vi "Draw Markers.vi"(7 "XYGraph in":refnum<vi>, 9 "Marker Options":T3={"Color"=16723218, "pen"={"Width"=2, "Style"=enum."Solid"}, "font"={"Font Name"="Arial", "Size"=16, "Strikeout?"=FALSE, "Italic?"=FALSE, "Underline?"=FALSE, "Outline?"=FALSE, "Shadow?"=FALSE, "Bold?"=FALSE, "FontColor"=0}, "caption"=""}, 10 "Marker":T1={"Type"=enum."vert", "X"=2.0, "Y"=2.0, "X2"=2.0, "Y2"=2.0, "Text"="Drag and click to\nposition a marker"}, 11 "picture":picture) -> (3 "new picture":picture)   [LabVIEW 2014, in "Graph Extensions.lvlib"]
doc: "Draw the appropriate line for markers, depending on the type"
uses:
  Graph Extensions.lvlib
  <vilib>/Utility/miscctls.llb/LVPoint32TypeDef.ctl
  controls/MarkerInfo.ctl
  controls/MarkerOptions.ctl
  controls/markerType.ctl
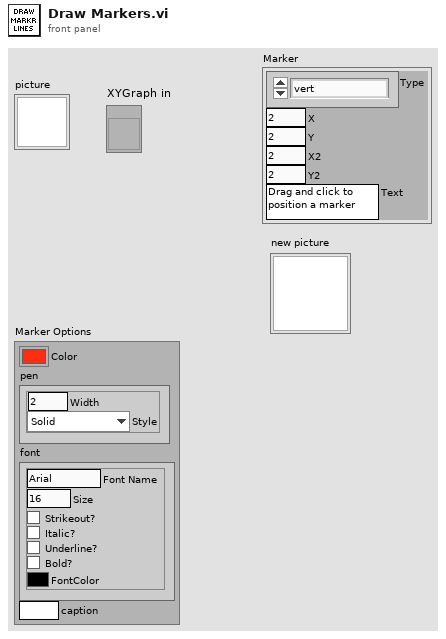
[diagram p1: front panel]
types:
  T1 = typedef "Graph Extensions.lvlib/MarkerInfo.ctl" = cluster{"Type":T2, "X":dbl, "Y":dbl, "X2":dbl, "Y2":dbl, "Text":string}
  T2 = typedef "Graph Extensions.lvlib/markerType.ctl" = enum16{"point", "arrow", "horiz", "vert", "vert range", "horiz range", "box"}
  T3 = typedef "Graph Extensions.lvlib/MarkerOptions.ctl" = cluster{"Color":u32, "pen":cluster{"Width":u16, "Style":enum32{"Solid", "Dash", "Dot", "DashDot", "DashDotDot"}}, "font":cluster{"Font Name":string, "Size":i16, "Strikeout?":bool, "Italic?":bool, "Underline?":bool, "Outline?":bool, "Shadow?":bool, "Bold?":bool, "FontColor":u32}, "caption":string}
  T4 = cluster{"Font Name:":string, "Size":i16, "Strikeout?":bool, "Italic?":bool, "Underline?":bool, "Outline?":bool, "Shadow?":bool, "Bold?":bool}
  T5 = enum16{"User-specified Font", "Application Font", "System Font", "Dialog Font"}
  T6 = typedef "LVPoint32TypeDef.ctl" = cluster{"Horizontal":i32, "Vertical":i32}
  T7 = typedef "LVRectTypeDef.ctl" = cluster{"Left":i16, "Top":i16, "Right":i16, "Bottom":i16}
  T8 = cluster{"Font Name":string, "Size":i16, "Strikeout?":bool, "Italic?":bool, "Underline?":bool, "Outline?":bool, "Shadow?":bool, "Bold?":bool, "FontColor":u32}
  T9 = cluster{"Width":u16, "Style":enum32{"Solid", "Dash", "Dot", "DashDot", "DashDotDot"}}
  T10 = cluster{"left":i16, "top":i16, "right":i16, "bottom":i16}
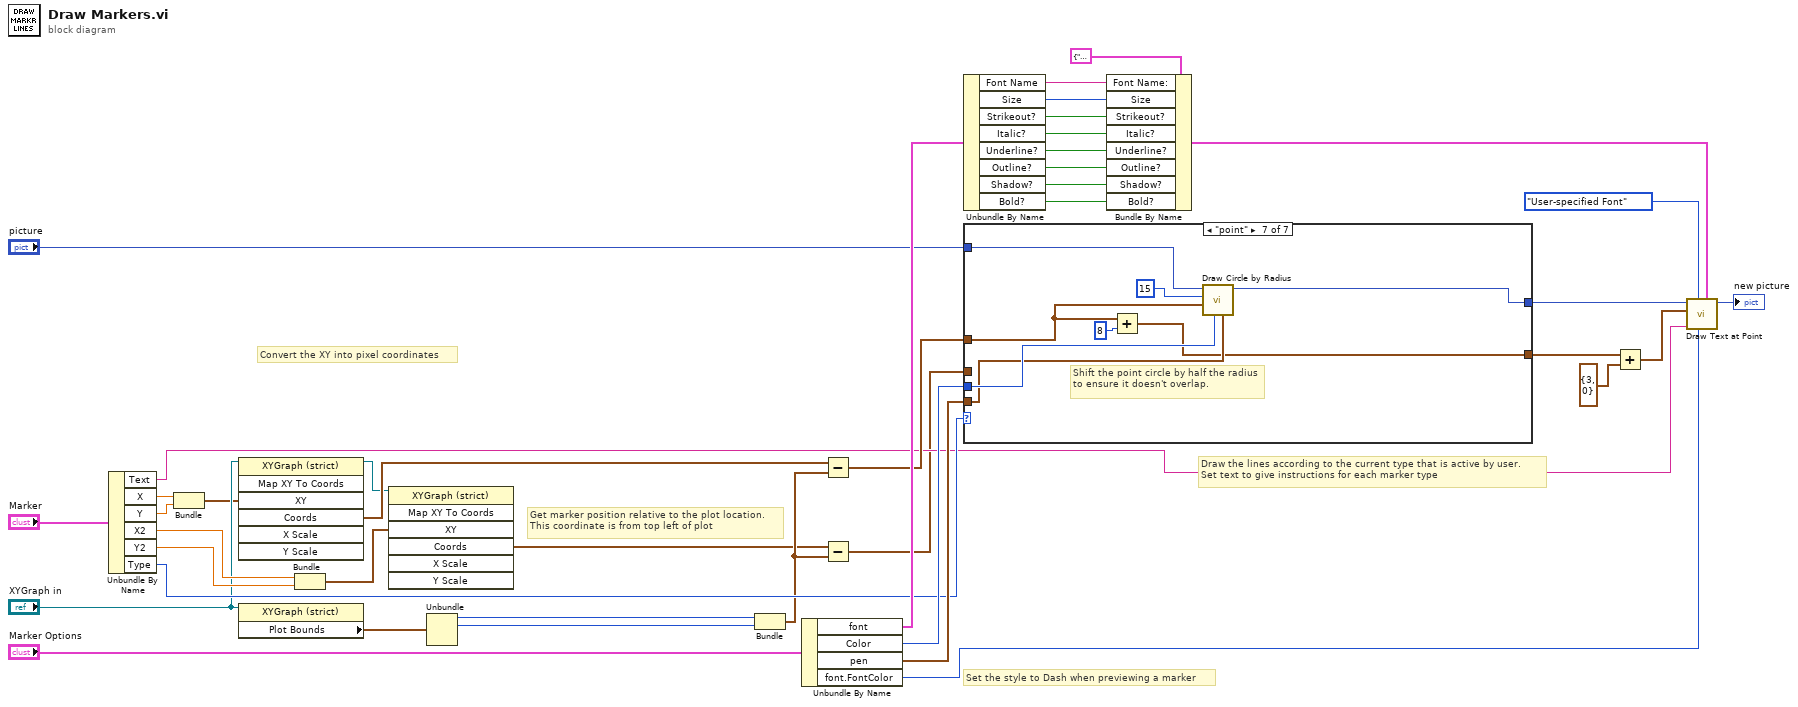
[diagram p0: block diagram]
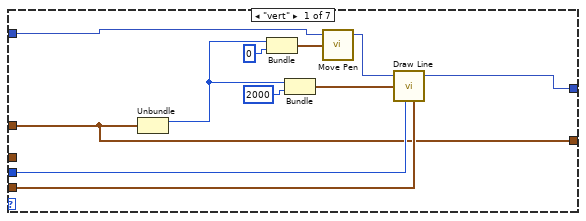
[diagram p2: hidden frame]
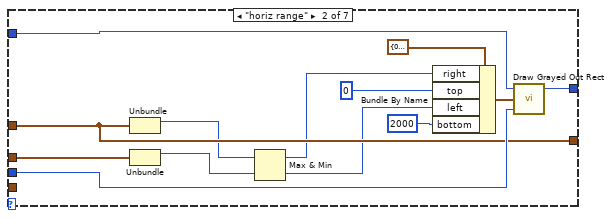
[diagram p3: hidden frame]
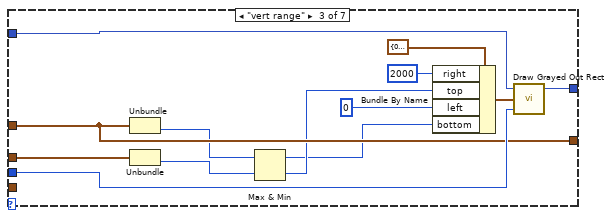
[diagram p4: hidden frame]
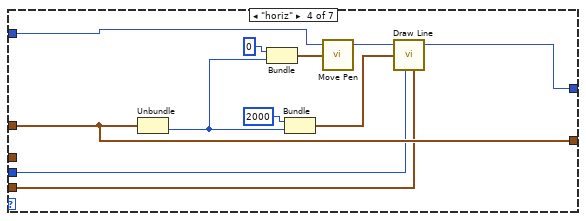
[diagram p5: hidden frame]
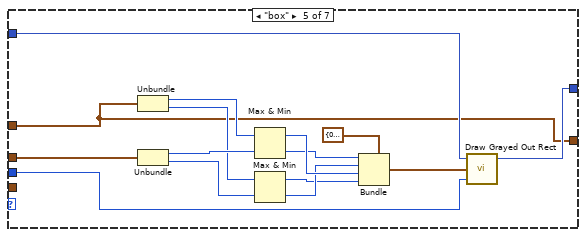
[diagram p6: hidden frame]
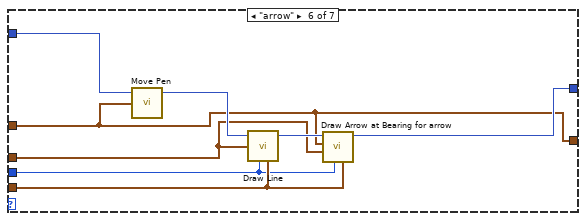
[diagram p7: hidden frame]
diagram:
  # "Convert the XY into pixel coordinates"
  # "Get marker position relative to the plot location.\nThis coordinate is from top left of plot"
  # "Set the style to Dash when previewing a marker"
  # "Draw the lines according to the current type that is active by user.\nSet text to give instructions for each marker type"
  n1 = Unbundle By Name("Marker") -> ("Text"=w11:string, "X"=w20:dbl, "Y"=w19:dbl, "X2"=w10:dbl, "Y2"=w9:dbl, "Type"=w12:T2)
  n2 = Bundle("X"=w20, "Y"=w19) -> (w5:cluster{"X":dbl, "Y":dbl})  [unwired: 1 in]
  n3 = invoke class="XYGraph (strict)" method="Map XY To Coords"(reference="XYGraph in", "XY"=w5) -> (reference out=w3:refnum<vi>, "Coords"=w4:T6)  [unwired: 5 in, 5 out]
  n4 = property on="Property Node" class="XYGraph (strict)"(reference="XYGraph in") -> ("Plot Bounds"=w15:T7)  [unwired: 1 in, 2 out]
  n5 = Bundle("X2"=w10, "Y2"=w9) -> (w2:cluster{"X2":dbl, "Y2":dbl})  [unwired: 1 in]
  n6 = invoke class="XYGraph (strict)" method="Map XY To Coords"(reference=w3, "XY"=w2) -> ("Coords"=w1:T6)  [unwired: 5 in, 6 out]
  n7 = Unbundle(w15) -> ("Left"=w16:i16, "Top"=w17:i16)  [unwired: 2 out]
  n8 = Bundle("Left"=w16, "Top"=w17) -> (w8:cluster{"Left":i16, "Top":i16})  [unwired: 1 in]
  n9 = Unbundle By Name("Marker Options") -> ("font"=w24:T8, "Color"=w26:u32, "pen"=w13:T9, "font.FontColor"=w37:u32)
  n10 = Subtract(x=w4, y=w8) -> (x-y=w14:T6)
  n11 = Subtract(x=w1, y=w8) -> (x-y=w7:T6)
  n12 = Unbundle By Name(w24) -> ("Font Name"=w35:string, "Size"=w34:i16, "Strikeout?"=w33:bool, "Italic?"=w32:bool, "Underline?"=w31:bool, "Outline?"=w30:bool, "Shadow?"=w29:bool, "Bold?"=w28:bool)
  n13 = case shown="\"point\"" w12 {
    tunnel: w14 -> [w42 w63 w76 w82 w90 w105 w115]
    tunnel: [w50 w65 w78 w88 w102 w109 w120] -> w39
    tunnel: "picture" -> [w45 w57 w72 w79 w104 w111 w116]
    tunnel: w26 -> [w44 w64 w77 w81 w103 w107 w119]
    tunnel: w13 -> [w43 _ _ w80 _ w108 w117]
    tunnel: [w42 w63 w76 w82 w90 w105 w113] -> w25
    tunnel: w7 -> [_ w58 w73 _ w99 w106 _]
    frame "vert" {
      n14 = Unbundle(w42) -> ("Horizontal"=w52:i32)  [unwired: 1 out]
      n15 = Bundle("Horizontal"=w52, "top"=i16 0) -> (w46:cluster{"Horizontal":i32, "top":i16})  [unwired: 1 in]
      n16 = Bundle("Horizontal"=w52, "top"=i16 2000) -> (w51:cluster{"Horizontal":i32, "top":i16})  [unwired: 1 in]
      n17 = call <vilib>:"Move Pen.vi"("new position"=w46, "picture"=w45) -> ("new picture"=w49:picture)  [unwired: 3 in]
      n18 = call <vilib>:"Draw Line.vi"("picture"=w49, "end point"=w51, "color(black)"=w44, "pen"=w43) -> ("new picture"=w50:picture)  [unwired: 5 in]
    }
    frame "horiz range" {
      n19 = Unbundle(w63) -> ("Horizontal"=w56:i32)  [unwired: 1 out]
      n20 = Unbundle(w58) -> ("Horizontal"=w55:i32)  [unwired: 1 out]
      n21 = Max & Min(x=w56, y=w55) -> (max(x,y)=w53:i32, min(x,y)=w54:i32)
      n22 = Bundle By Name(cluster=T10 {"left"=0, "top"=0, "right"=0, "bottom"=0} ("rect"), "right"=w53, "top"=i16 0, "left"=w54, "bottom"=i16 2000) -> (w61:T10)
      n23 = call <vilib>:"Draw Grayed Out Rect.vi"("color(black)"=w64, "rect"=w61, "picture"=w57) -> ("new picture"=w65:picture)  [unwired: 2 in]
    }
    frame "vert range" {
      n24 = Unbundle(w76) -> ("Vertical"=w71:i32)  [unwired: 1 out]
      n25 = Unbundle(w73) -> ("Vertical"=w70:i32)  [unwired: 1 out]
      n26 = Max & Min(x=w71, y=w70) -> (max(x,y)=w66:i32, min(x,y)=w67:i32)
      n27 = Bundle By Name(cluster=T10 {"left"=0, "top"=0, "right"=0, "bottom"=0} ("rect"), "right"=i16 2000 ("top"), "top"=w67, "left"=i16 0 ("bottom"), "bottom"=w66) -> (w74:T10)
      n28 = call <vilib>:"Draw Grayed Out Rect.vi"("color(black)"=w77, "rect"=w74, "picture"=w72) -> ("new picture"=w78:picture)  [unwired: 2 in]
    }
    frame "horiz" {
      n29 = Unbundle(w82) -> ("Vertical"=w84:i32)  [unwired: 1 out]
      n30 = Bundle("top"=i16 0, "Vertical"=w84) -> (w86:cluster{"top":i16, "Vertical":i32})  [unwired: 1 in]
      n31 = Bundle("top"=i16 2000, "Vertical"=w84) -> (w89:cluster{"top":i16, "Vertical":i32})  [unwired: 1 in]
      n32 = call <vilib>:"Move Pen.vi"("new position"=w86, "picture"=w79) -> ("new picture"=w87:picture)  [unwired: 3 in]
      n33 = call <vilib>:"Draw Line.vi"("picture"=w87, "end point"=w89, "color(black)"=w81, "pen"=w80) -> ("new picture"=w88:picture)  [unwired: 5 in]
    }
    frame "box" {
      n34 = Unbundle(w90) -> ("Horizontal"=w98:i32, "Vertical"=w94:i32)
      n35 = Unbundle(w99) -> ("Horizontal"=w97:i32, "Vertical"=w93:i32)
      n36 = Max & Min(x=w98, y=w97) -> (max(x,y)=w96:i32, min(x,y)=w95:i32)
      n37 = Max & Min(x=w94, y=w93) -> (max(x,y)=w91:i32, min(x,y)=w92:i32)
      n38 = Bundle(cluster=T10 {"left"=0, "top"=0, "right"=0, "bottom"=0} ("rect"), "left"=w95, "top"=w92, "right"=w96, "bottom"=w91) -> (w101:T10)
      n39 = call <vilib>:"Draw Grayed Out Rect.vi"("color(black)"=w103, "rect"=w101, "picture"=w104) -> ("new picture"=w102:picture)  [unwired: 2 in]
    }
    frame "arrow" {
      n40 = call <vilib>:"Move Pen.vi"("new position"=w105, "picture"=w111) -> ("new picture"=w112:picture)  [unwired: 3 in]
      n41 = call <vilib>:"Draw Line.vi"("picture"=w112, "end point"=w106, "color(black)"=w107, "pen"=w108) -> ("new picture"=w110:picture)  [unwired: 5 in]
      n42 = call "Draw Arrow at Bearing for arrow.vi"("pen"=w108, "color(black)"=w107, "P2"=w106, "P1"=w105, "new picture in"=w110) -> ("new picture out"=w109:picture)  [unwired: 6 in]
    }
    frame "point" {
      # "Shift the point circle by half the radius to ensure it doesn't overlap."
      n43 = Add(x=w115, y=8 ("Horizontal")) -> (x+y=w113:T6)
      n44 = call <vilib>:"Draw Circle by Radius.vi"("pen"=w117, "color(black)"=w119, "pixel center"=w115, "radius"=i16 15, "picture"=w116) -> ("new picture"=w120:picture)  [unwired: 6 in]
    }
  }
  n45 = Bundle By Name(cluster=T4 {"Font Name:"="", "Size"=12, "Strikeout?"=FALSE, "Italic?"=FALSE, "Underline?"=FALSE, "Outline?"=FALSE, "Shadow?"=FALSE, "Bold?"=FALSE} ("[user-specified font]"), "Font Name:"=w35, "Size"=w34, "Strikeout?"=w33, "Italic?"=w32, "Underline?"=w31, "Outline?"=w30, "Shadow?"=w29, "Bold?"=w28) -> (w27:T4)
  n46 = Add(x=w25, y=T6 {"Horizontal"=3, "Vertical"=0}) -> (x+y=w40:T6)
  n47 = call <vilib>:"Draw Text at Point.vi"("[user-specified font]"=w27, "text color(black)"=w37, "desired font(Application)"=T5."User-specified Font", "text"=w11, "origin"=w40, "picture"=w39) -> ("new picture"=→"new picture":picture)  [unwired: 4 in, 1 out]
